vi "DrawLines.vi"(8 "error in (no error)":errorcluster, 11 "Menu in":refnum<class "Menu.lvclass">) -> (0 "error out":errorcluster, 3 "Menu out":refnum<class "Menu.lvclass">)   [LabVIEW 2019, in "RT_Game.lvlib" / "Menu.lvclass"]
uses:
  Menu.lvclass
  C:/Users/FreshBob/Dropbox/VIs/myRIO_GameConsole/RT/RT_Game/Game/Game.lvclass
  Game/Coordinate.ctl
  Menu.lvclass/Menu.ctl
  Game/Game.lvclass
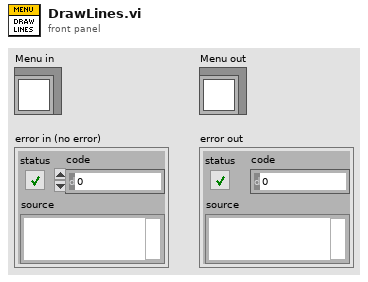
[diagram p1: front panel]
types:
  T1 = typedef "RT_Game.lvlib/Game.lvclass/Coordinate.ctl" = cluster{"x":dbl, "y":dbl}
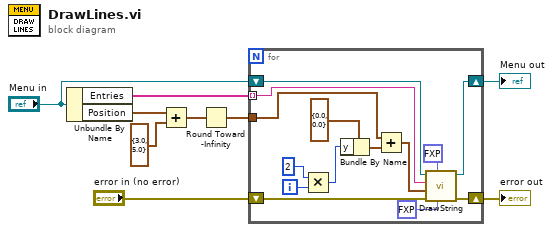
[diagram p0: block diagram]
diagram:
  n1 = Unbundle By Name("Menu in") -> ("Entries"=w5:string[], "Position"=w4:T1)
  n2 = Add(x=w4, y=T1 {"x"=3.0, "y"=5.0}) -> (x+y=w3:T1)
  n3 = Round Toward -Infinity(1:w3) -> (0:w1:T1)
  n4 = for {
    shift-right: [w22] -> w8
    shift-left: "error in (no error)" -> [w23]
    shift-right: [w21] -> w7
    shift-left: "Menu in" -> [w20]
    tunnel: w5 -> [w19] mode=indexing
    tunnel: w1 -> [w18]
    i -> [w14]
    n5 = Multiply(x=2, y=w14) -> (x*y=w13:i32)
    n6 = Bundle By Name(cluster=T1 {"x"=0.0, "y"=0.0} ("y"), "y"=w13) -> (w15:T1)
    n7 = Add(x=w18, y=w15) -> (x+y=w17:T1)
    n8 = call "DrawString.vi"("ColorToReplace (7=white)"=fxp<+,3,3> 5.0, "Color (7=white)"=fxp<+,3,3> 1.0, "error in (no error)"=w23, "Coordinate"=w17, "String"=w19, "RT_Game.lvlib:Game.lvclass"=w20) -> ("error out"=w22:errorcluster, "RT_Game.lvlib:Game.lvclass 2"=w21:refnum<class "Menu.lvclass">)  [unwired: 4 in]
  }
  "error out" <- w8
  "Menu out" <- w7
